vi "ESR Scanner - pulsed optimizer.vi"(0 "ESR Parameters":T3={"Window 1 time (s)"=0.012, "Window 2 time (s)"=5e-06, "Window 3 time (s) "=0.02, "Window 4 time (s)"=5e-07, "Window 4 channels"=[TRUE, FALSE, FALSE, TRUE], "Window 3 channels"=[TRUE, FALSE, TRUE, TRUE], "Window 2 channels"=[TRUE, FALSE, FALSE, TRUE], "Window 1 channels"=[TRUE, TRUE, FALSE, TRUE], "Path to ESR Burner"=path "C:/Users/Loncar/Desktop/ESR VIs - Srujan/Sam Kim/PB/ESRFreq.exe"}, 1 "MW start freq (GHz)":dbl=2.84, 2 "MW stop freq (GHz)":dbl=2.9, 3 "# freq points":i32=61, 4 "# scans before track":i32=50, 5 "#scan iterations":i32=50, 6 "IntGraph Refnum":refnum<vi>, 7 "Optimize Parameters":T4={"Volt Step"={"X"=0.01, "Y"=0.01, "Z"=0.0}, "Num Iterations"=1, "Dwell Time (ms)"=100, "Volts Range"={"X"=0.1, "Y"=0.1, "Z"=0.0}, "Method"={"X"=enum."Max", "Y"=enum."Max", "Z"=enum."Max"}} {"Volts Range"."Z" min=0.0; "Volts Range"."Y" min=0.0; "Volts Range"."X" min=0.0; "Dwell Time (ms)" min=0; "Num Iterations" min=1 step=1; "Volt Step"."Z" min=1e-05; "Volt Step"."Y" min=1e-06; "Volt Step"."X" min=1e-06}, 8 "XY Graph Refnum":refnum<vi>, 9 "ESR Post-Processing Parameters":T1={"Cut-off Threshhold"=2.0, "Processing Type"=enum."Off"}, 14 "Save avg spectrum data to spreadsheet?":bool, 15 "Path for avg spectrum spreadsheet":path=path "C:/experiment/data/may_15_2012/SIL1_NV1_pippin_uW_off", 16 "Save avg spectrum graph?":bool, 17 "Path for avg spectrum graph":path=path "C:/experiment/data/may_15_2012/SIL1_NV1_pippin_uW_off") -> ()   [LabVIEW 2012]
uses:
  Strict Type Def - Optimize Parameters Cluster.ctl
  ESR Window Parameters.ctl
  ESR Processing Params.ctl
  ESR Processing State.ctl
  <vilib>/DAQmx/read.llb/DAQmx Read (Counter 1D U32 1Chan NSamp).vi
  Channels.vi
  <vilib>/DAQmx/miscellaneous.llb/DAQmx Fill In Error Info.vi
  Global Vars.vi
  <vilib>/Analysis/baseanly.llb/Mean (DBL).vi
  <vilib>/Utility/file.llb/Write To Spreadsheet File (DBL).vi
  <vilib>/Analysis/NI_AALBase.lvlib
panel:
  out "Counts vs. frequency before processing":i32[][](graph)
  out "Counts vs. frequency":i32[][](graph)
  out "Avg ESR spectrum":cluster{"Y":dbl[], "Y":dbl[]}[](graph)
  # "Note:\nThis is not a standalone program. It is called from ScannerUI"
  # "Default PB connections:\nPB0 - MW switch\nPB1 - MW freq step\nPB2 - Counter sample clk\nPB3 - Green AOM"
  # "VI for ESR spectrum measurement\n08/26/2013, Srujan Meesala\n12/18/2013, Samuel Kim"
  # "Stop experiment and\nreset PulseBlaster"
  # "* <data>"
  # "MW freq step\ndwell time"
  # "MW freq step"
  # "Wait"
  # "Fluorescence\ncounting"
  # "Ctr sample clk"
  # "Wait"
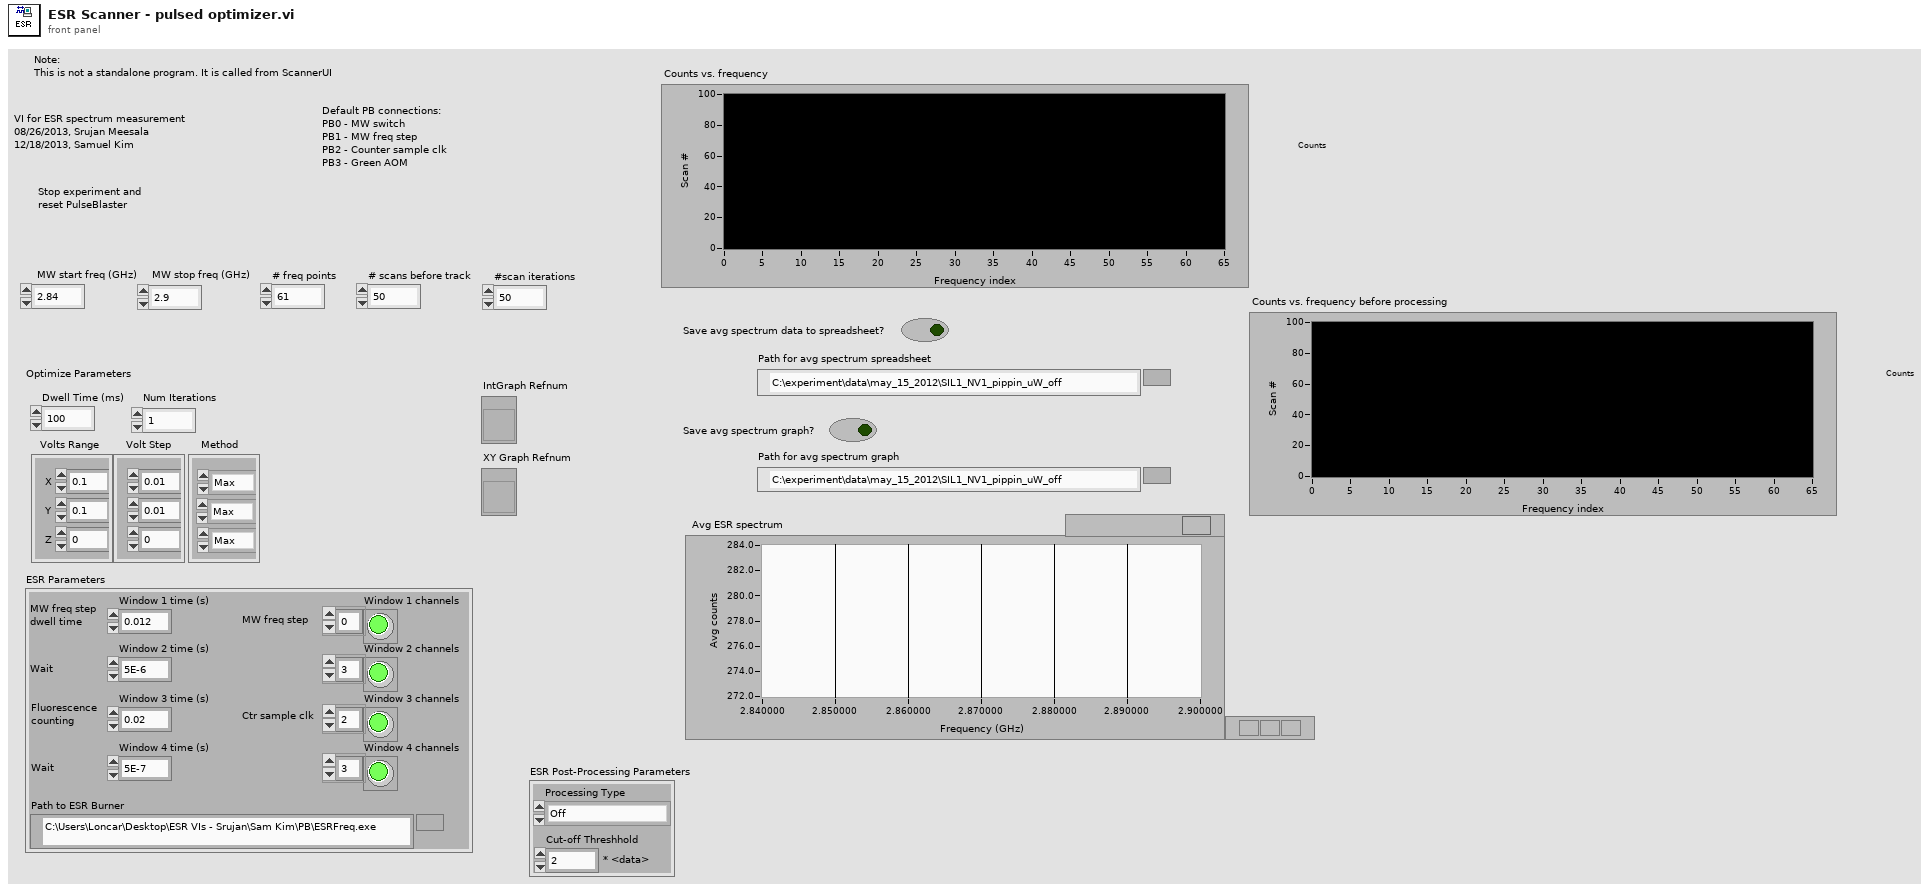
[diagram p1: front panel]
types:
  T1 = typedef "ESR Processing Params.ctl" = cluster{"Cut-off Threshhold":dbl, "Processing Type":T2}
  T2 = typedef "ESR Processing State.ctl" = enum16{"Off", "Remove Outlier Scan", "Remove Outlier Data"}
  T3 = typedef "ESR Window Parameters.ctl" = cluster{"Window 1 time (s)":dbl, "Window 2 time (s)":dbl, "Window 3 time (s) ":dbl, "Window 4 time (s)":dbl, "Window 4 channels":bool[], "Window 3 channels":bool[], "Window 2 channels":bool[], "Window 1 channels":bool[], "Path to ESR Burner":path}
  T4 = typedef "Strict Type Def - Optimize Parameters Cluster.ctl" = cluster{"Volt Step":cluster{"X":dbl, "Y":dbl, "Z":dbl}, "Num Iterations":i32, "Dwell Time (ms)":i32, "Volts Range":cluster{"X":dbl, "Y":dbl, "Z":dbl}, "Method":cluster{"X":enum16{"Max", "Gaussian"}, "Y":enum16{"Max", "Gaussian"}, "Z":enum16{"Max", "Gaussian"}}}
  T5 = typedef "imagedata.ctl" = cluster{"image type":i32, "image depth":i32, "image":u8[], "mask":u8[], "colors":u32[], "Rectangle":cluster{"left":i16, "top":i16, "right":i16, "bottom":i16}}
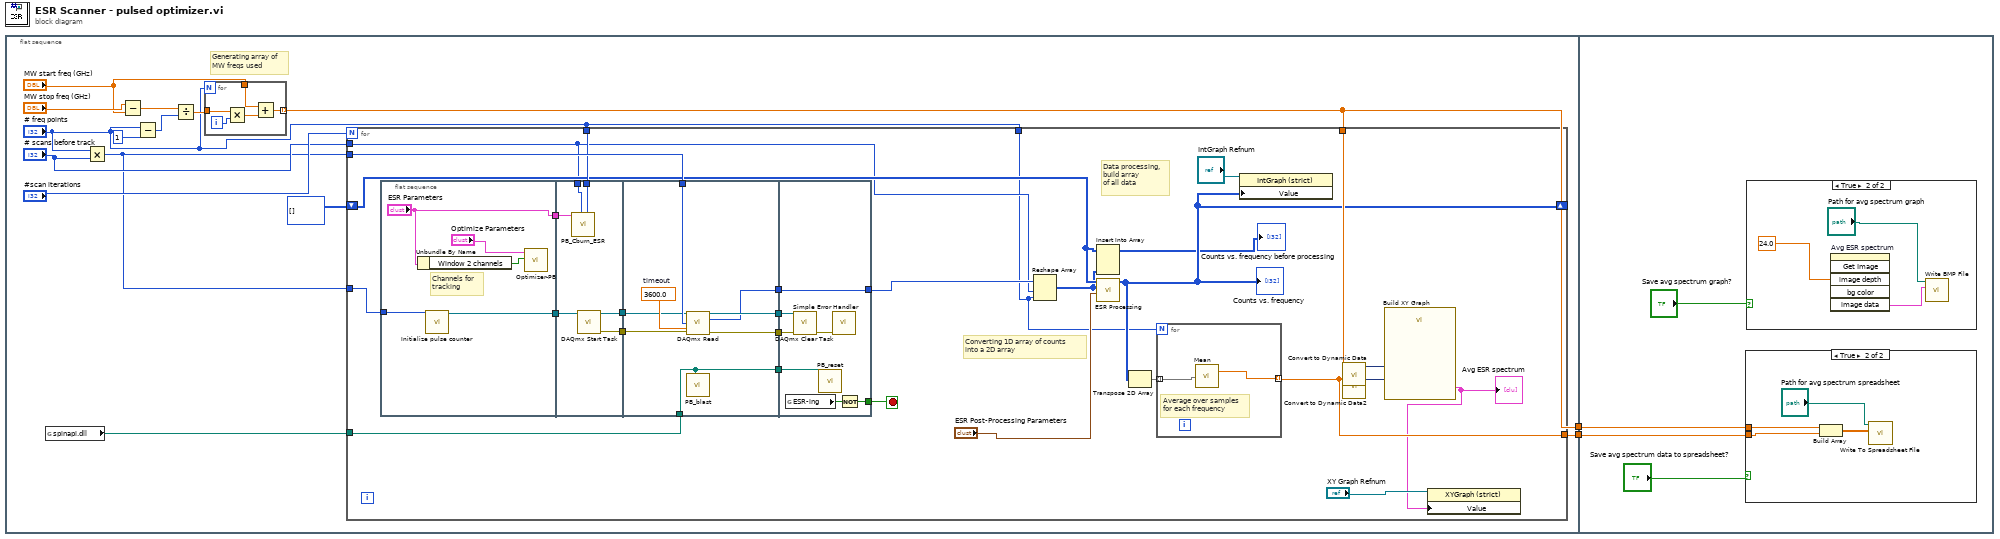
[diagram p0: block diagram]
diagram:
  n1 = flat-sequence {
    tunnel: [w8] -> w2
    tunnel: [w7] -> w1
    tunnel: w2 -> [w80]
    tunnel: w1 -> [w79]
    frame #0 {
      # "Generating array of\nMW freqs used"
      n2 = global read "Channels.vi" "spinapi.dll"() -> (w5:path)
      n3 = Multiply(x="# freq points", y="# scans before track") -> (x*y=w3:i32)
      n4 = Subtract(x="MW stop freq (GHz)", y="MW start freq (GHz)") -> (x-y=w14:dbl)
      n5 = Subtract(x="# freq points", y=u32 1 ("Reset Count")) -> (x-y=w15:u32)
      n6 = Divide(x=w14, y=w15) -> (x/y=w12:dbl)
      n7 = for {
        N: "# freq points" -> [_]
        tunnel: w12 -> [w77]
        tunnel: "MW start freq (GHz)" -> [w75]
        tunnel: [w74] -> w8 mode=indexing
        i -> [w78]
        n8 = Multiply(x=w77, y=w78) -> (x*y=w76:dbl)
        n9 = Add(x=w75, y=w76) -> (x+y=w74:dbl)
      }
      n10 = for {
        N: "#scan iterations" -> [_]
        tunnel: w5 -> [w25]
        tunnel: w3 -> [w45]
        tunnel: "# scans before track" -> [w19]
        tunnel: "# freq points" -> [w18]
        shift-right: [w34] -> _
        shift-left: i32[][] [] ("Flourescence Data") -> [w22]
        tunnel: w8 -> [w37]
        tunnel: [w36] -> w7
        tunnel: "# freq points" -> [w30]
        tunnel: w3 -> [w27]
        stop <- w24 stop-if-true
        # "Data processing,\nbuild array\nof all data"
        # "Converting 1D array of counts \ninto a 2D array"
        n11 = flat-sequence {
          tunnel: ["ESR Parameters"] -> w31
          tunnel: w27 -> [w51]
          tunnel: [w50] -> w26
          tunnel: w31 -> [w53]
          tunnel: w19 -> [w55]
          tunnel: w30 -> [w54]
          tunnel: [w58] -> w29
          tunnel: [w57] -> w28
          tunnel: w26 -> [w56]
          tunnel: w45 -> [w65]
          tunnel: w25 -> [w62]
          tunnel: [w64] -> w44
          tunnel: [w63] -> w43
          tunnel: [w62] -> w42
          tunnel: [w59] -> w38
          tunnel: w29 -> [w61]
          tunnel: w28 -> [w60]
          tunnel: w44 -> [w70]
          tunnel: w43 -> [w71]
          tunnel: w42 -> [w73]
          tunnel: [w72] -> w20
          tunnel: w38 -> [w72]
          tunnel: [w67] -> w24
          frame #0 {
            # "Channels for\ntracking"
            n12 = Unbundle By Name("ESR Parameters") -> ("Window 2 channels"=w49:bool[])
            n13 = call "Initialize pulse counter.vi"("Samples per channel"=w51) -> ("DAQmx Task Name"=w50:refnum<k21>)  [unwired: 9 in, 1 out]
            n14 = call "Optimizer-PB.vi"("Optimize active channels"=w49, "Optimize Parameters"="Optimize Parameters") -> ()  [unwired: 8 in, 2 out]
          }
          frame #1 {
            n15 = call "PB_Cburn_ESR.vi"("# freq points"=w54, "# scans before track"=w55, "ESR Parameters"=w53) -> ()  [unwired: 9 in]
            n16 = call <vilib>:"DAQmx Start Task.vi"("task/channels in"=w56) -> ("task out"=w58:refnum<k21>, "error out"=w57:errorcluster)  [unwired: 13 in]
          }
          frame #2 {
            w66 = 3600.0  # timeout
            n17 = call-poly <vilib>:"DAQmx Read.vi"("task/channels in"=w61, "number of samples per channel"=w65, "timeout"=w66, "error in"=w60) -> ("task out"=w63:refnum<k21>, "data"=w59:u32[], "error out"=w64:errorcluster)  [unwired: 9 in]
            n18 = call "PB_blast.vi"("Path to spinapi.dll"=w62) -> ()  [unwired: 7 in]
          }
          frame #3 {
            n19 = global read "Global Vars.vi" "ESR-ing"() -> (w68:bool)
            n20 = call <vilib>:"DAQmx Clear Task.vi"("task in"=w71, "error in"=w70) -> ("error out"=w69:errorcluster)  [unwired: 13 in]
            n21 = call "PB_reset.vi"("Path to spinapi.dll"=w73) -> ()  [unwired: 7 in]
            n22 = call <vilib>:"Simple Error Handler.vi"("error in (no error)"=w69) -> ()  [unwired: 4 in, 5 out]
            n23 = Not(x=w68) -> (.not. x?=w67:bool)
          }
        }
        n24 = Reshape Array(w20, w19, w18) -> (w17:u32[][])
        n25 = Insert Into Array(array=w22, new element=w17) -> (→"Counts vs. frequency before processing":i32[][])  [unwired: 2 in]
        n26 = call "ESR Processing.vi"("ESR Post-Processing Parameters"="ESR Post-Processing Parameters", "Array"=w17, "Flourescence Data in"=w22) -> ("Flourescence Data out"=w34:i32[][])  [unwired: 8 in]
        "Counts vs. frequency" <- w34
        n27 = Transpose 2D Array(2D array=w34) -> (transposed array=w39:i32[][])
        n28 = for {
          N: w18 -> [_]
          tunnel: [w47] -> w36 mode=indexing
          tunnel: w39 -> [w46] mode=indexing
          # "Average over samples\nfor each frequency"
          n29 = call-poly <vilib>:"Mean.vi"("X"=w46) -> ("mean"=w47:dbl)  [unwired: 1 out]
        }
        n30 = property class="IntGraph (strict)"(reference="IntGraph Refnum", "Value"=w34) -> ()  [unwired: 1 in, 2 out]
        n31 = call "Convert to Dynamic Data"("Array"=w37) -> ("Dynamic Data Type"=w41:dynamicdata)  [unwired: 3 in]
        n32 = call "Convert to Dynamic Data2"("Array"=w36) -> ("Dynamic Data Type"=w40:dynamicdata)  [unwired: 3 in]
        n33 = call "Build XY Graph"("Y Input"=w40, "X Input"=w41) -> ("XY Graph"=w32:cluster{"Y":dbl[], "Y":dbl[]}[])  [unwired: 3 in, 6 out]
        "Avg ESR spectrum" <- w32
        n34 = property class="XYGraph (strict)"(reference="XY Graph Refnum", "Value"=w32) -> ()  [unwired: 1 in, 2 out]
      }
    }
    frame #1 {
      n35 = case shown="True" "Save avg spectrum data to spreadsheet?" {
        tunnel: w80 -> [_ w84]
        tunnel: w79 -> [_ w83]
        frame False {
        }
        frame True {
          n36 = Build Array(w84, w83) -> (w85:dbl[][])
          n37 = call-poly <vilib>:"Write To Spreadsheet File.vi"("2D data"=w85, "file path (dialog if empty)"="Path for avg spectrum spreadsheet") -> ()  [unwired: 6 in, 1 out]
        }
      }
      n38 = case shown="True" "Save avg spectrum graph?" {
        frame False {
        }
        frame True {
          n39 = invoke on="Avg ESR spectrum" class="XYGraph (strict)" method="Get Image"("image depth"=24.0 ("Initial Delay")) -> ("image data"=w87:T5)  [unwired: 5 in, 5 out]
          n40 = call <vilib>:"Write BMP File.vi"("image data"=w87, "path to BMP file"="Path for avg spectrum graph") -> ()  [unwired: 8 in, 2 out]
        }
      }
    }
  }
